vi "ConfigAcq.vi"(8 "error in (no error)":errorcluster, 11 "NiDaqMx in":refnum<class "NiDaqMx.lvclass">) -> (0 "error out":errorcluster, 3 "NiDaqMx out":refnum<class "NiDaqMx.lvclass">)   [LabVIEW 2014, in "DigitizerPlugins.lvlib" / "NiDaqMx.lvclass"]
uses:
  NiDaqMx.lvclass
  DigitizerBaseClass/DigitizerBase.lvclass/DigitizerBase.ctl
  NiDaqMx.lvclass/NiDaqMx.ctl
  DigitizerBaseClass/Accessors/Read InstRef.vi
  Accessors/Read SampleClock.vi
  DigitizerBaseClass/Accessors/Read Acquisition.vi
  DigitizerBaseClass/Accessors/Write InstRef.vi
  <vilib>/Utility/error.llb/Error Cluster From Error Code.vi
  <vilib>/DAQmx/configure/timing.llb/DAQmx Timing (Sample Clock).vi
  <vilib>/ErrorRing/Error Ring.xnode
  <resource>/objmgr/daqmx.rc
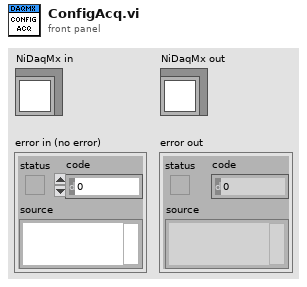
[diagram p1: front panel]
types:
  T1 = typedef "DigitizerPlugins.lvlib/NiDaqMx.lvclass/SampleClock.ctl" = cluster{"Type":enum16{"NULL", "Onboard", "External", "Software", "Interval"}, "Source":string, "TimebaseRate":dbl, "sample mode":i32}
  T2 = typedef "DigitizerPlugins.lvlib/DigitizerBase.lvclass/Acquisition.ctl" = cluster{"SampleRate":dbl, "RecordSize":i32, "NumRecords":i32, "SampleMode":i32, "Timeout (ms)":i32}
  T3 = enum16{"NULL", "Onboard", "External", "Software", "Interval"}
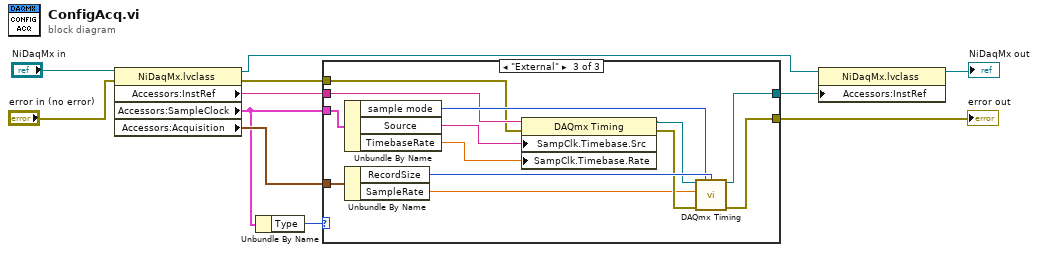
[diagram p0: block diagram]
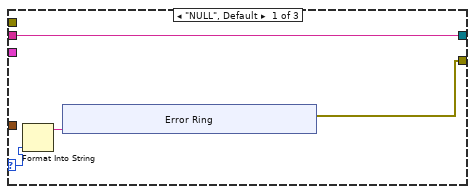
[diagram p2: hidden frame]
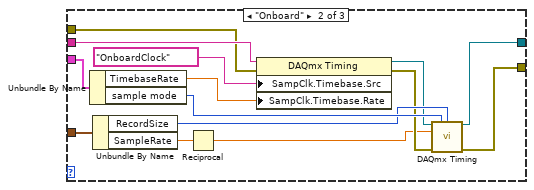
[diagram p3: hidden frame]
diagram:
  n1 = property class="NiDaqMx.lvclass"(reference="NiDaqMx in", error in="error in (no error)") -> (reference out=w7:refnum<class "NiDaqMx.lvclass">, error out=w3:errorcluster, "Accessors:InstRef"=w6:string, "Accessors:SampleClock"=w4:T1, "Accessors:Acquisition"=w5:T2)
  n2 = Unbundle By Name(w4) -> ("Type"=w9:T3)
  n3 = case shown="\"External\"" w9 {
    selector: w9 -> [w14 _ _]
    tunnel: [w13 w23 w38] -> w8
    tunnel: w6 -> [w12 w34 w44]
    tunnel: w5 -> [_ w31 w49]
    tunnel: w4 -> [_ w36 w47]
    tunnel: w3 -> [_ w33 w41]
    tunnel: [w12 w24 w39] -> w1
    frame "NULL", Default {
      n4 = Format Into String(w14) -> (resulting string=w15:string)  [unwired: 3 in, 1 out]
      n5 = xnode "Error Ring"("parameter 0"=w15) -> ("error out"=w13:errorcluster)
    }
    frame "Onboard" {
      n6 = Unbundle By Name(w36) -> ("TimebaseRate"=w35:dbl, "sample mode"=w29:i32)
      n7 = Unbundle By Name(w31) -> ("RecordSize"=w28:i32, "SampleRate"=w30:dbl)
      n8 = Reciprocal(x=w30) -> (1/x=w25:dbl)
      n9 = property class="DAQmx Timing"(reference=w34, error in=w33, "SampClk.Timebase.Src"=tag "OnboardClock", "SampClk.Timebase.Rate"=w35) -> (reference out=w27:refnum<k21>, error out=w26:errorcluster)
      n10 = call-poly <vilib>:"DAQmx Timing.vi"("task/channels in"=w27, "sample mode"=w29, "samples per channel"=w28, "rate"=w25, "error in"=w26) -> ("task out"=w24:refnum<k21>, "error out"=w23:errorcluster)  [unwired: 9 in]
    }
    frame "External" {
      n11 = Unbundle By Name(w47) -> ("sample mode"=w46:i32, "Source"=w43:string, "TimebaseRate"=w42:dbl)
      n12 = Unbundle By Name(w49) -> ("RecordSize"=w48:i32, "SampleRate"=w37:dbl)
      n13 = property class="DAQmx Timing"(reference=w44, error in=w41, "SampClk.Timebase.Src"=w43, "SampClk.Timebase.Rate"=w42) -> (reference out=w45:refnum<k21>, error out=w40:errorcluster)
      n14 = call-poly <vilib>:"DAQmx Timing.vi"("task/channels in"=w45, "sample mode"=w46, "samples per channel"=w48, "rate"=w37, "error in"=w40) -> ("task out"=w39:refnum<k21>, "error out"=w38:errorcluster)  [unwired: 9 in]
    }
  }
  "error out" <- w8
  n15 = property class="NiDaqMx.lvclass"(reference=w7, "Accessors:InstRef"=w1) -> (reference out=→"NiDaqMx out":refnum<class "NiDaqMx.lvclass">)  [unwired: 1 in, 1 out]
